vi "C-885 Chassis Engine.vi"() -> ()   [LabVIEW 2016]
uses:
  Stages Controls/Stage Notifier Element.ctl
  Stages Controls/Stage Actions.ctl
  Stages Controls/Stage Status.ctl
  C-885 Type Defs/C-885 Chassis Status.ctl
  PI GCS2 DLL/PI_GCS2_DLL_x64.dll
panel:
  in  "QUIT":bool
  in  "Abort":bool
  out "C-885 Found":bool
  out "Number Connected":i32
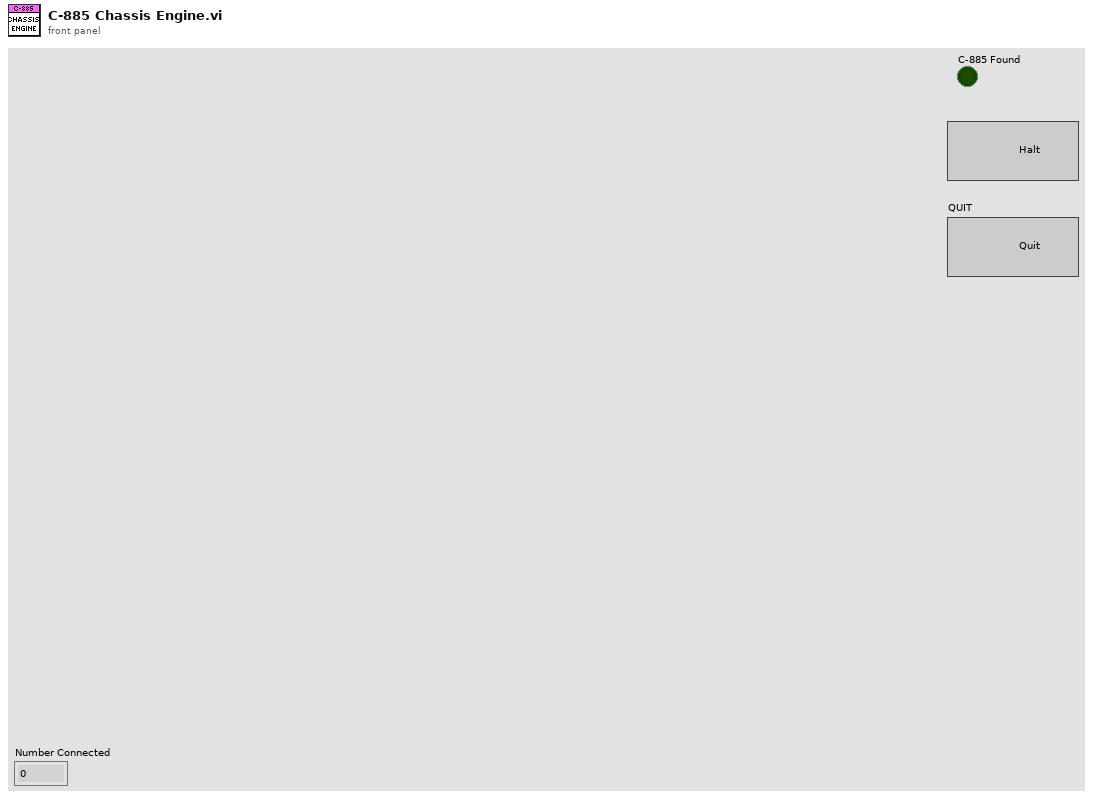
[diagram p1: front panel]
types:
  T1 = typedef "C-885 Chassis Status.ctl" = enum16{"Avalible", "Busy", "Halt"}
  T2 = typedef "Stage Notifier Element.ctl" = cluster{"Action":T3, "Axis":bool[], "Setpoint":dbl[], "Velocity":dbl, "Cmd Recvd?":bool, "Position":dbl[], "Status":T4, "Misc":variant}
  T3 = typedef "Stage Actions.ctl" = enum16{"Get Position", "MVR", "MOVE", "HALT", "ONTARGET", "ERROR", "REFERENCE", "INIT", "VELOCITY", "STATUS", "EXIT", "HOME", "ZEROPOS", "NANOPOS", "ANALOG", "QUIT"}
  T4 = typedef "Stage Status.ctl" = enum16{"Error", "Abort", "Busy", "On Target"}
  T5 = enum32{"Invalid", "Standard", "Closed", "Hidden", "Minimized", "Maximized"}
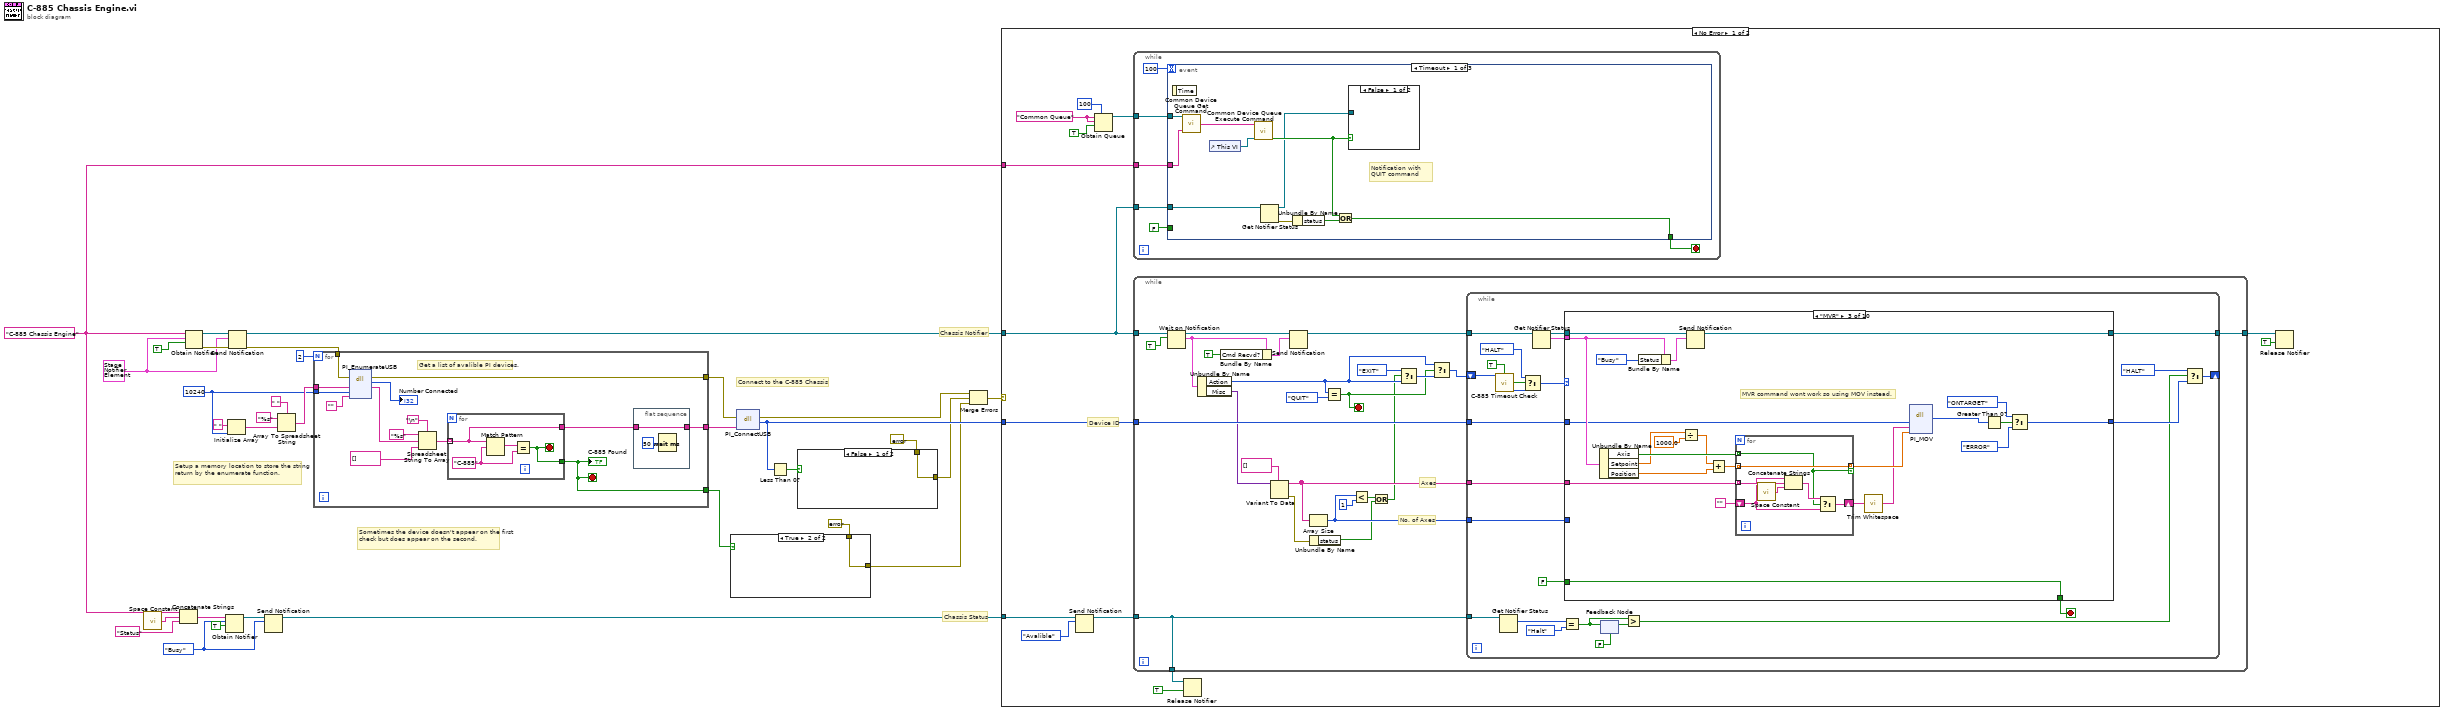
[diagram p0: block diagram]
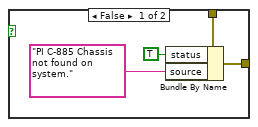
[diagram p2: hidden frame]
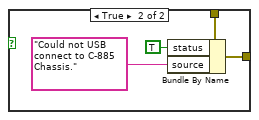
[diagram p3: hidden frame]
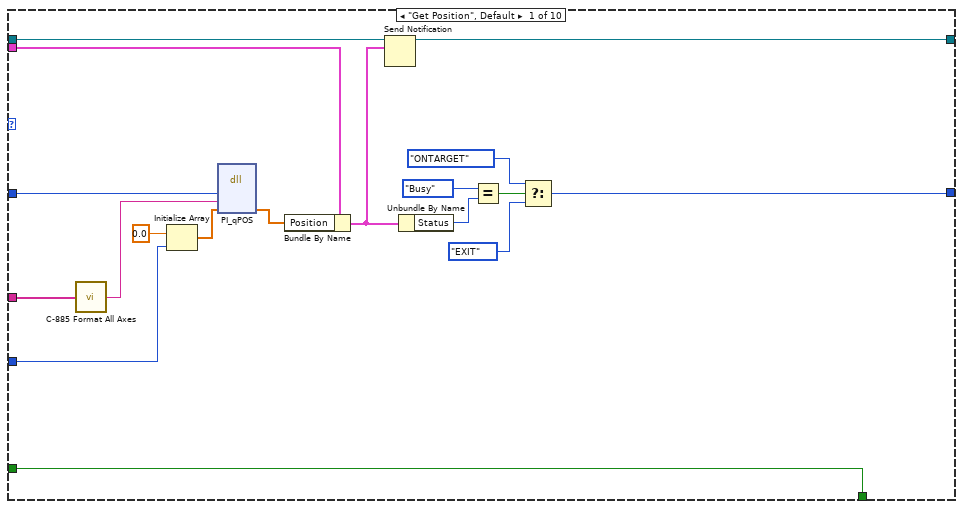
[diagram p4: hidden frame]
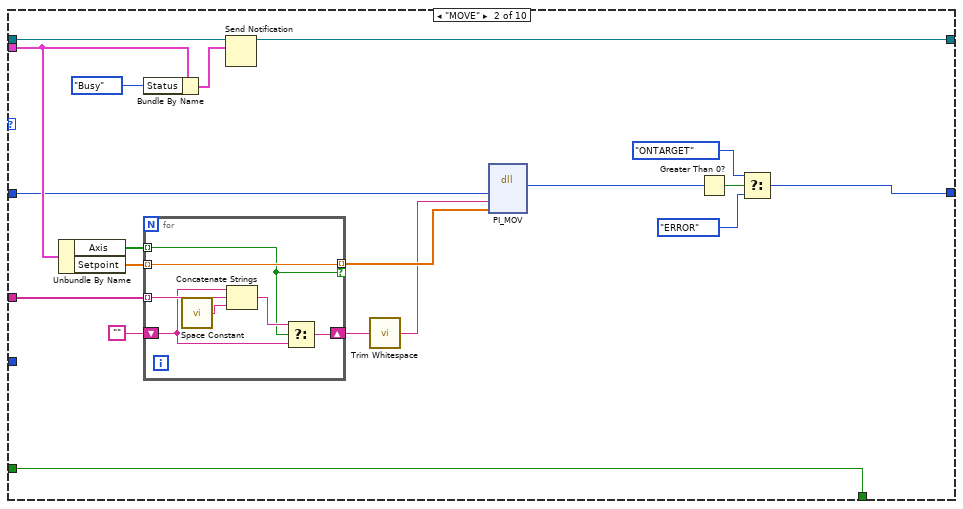
[diagram p5: hidden frame]
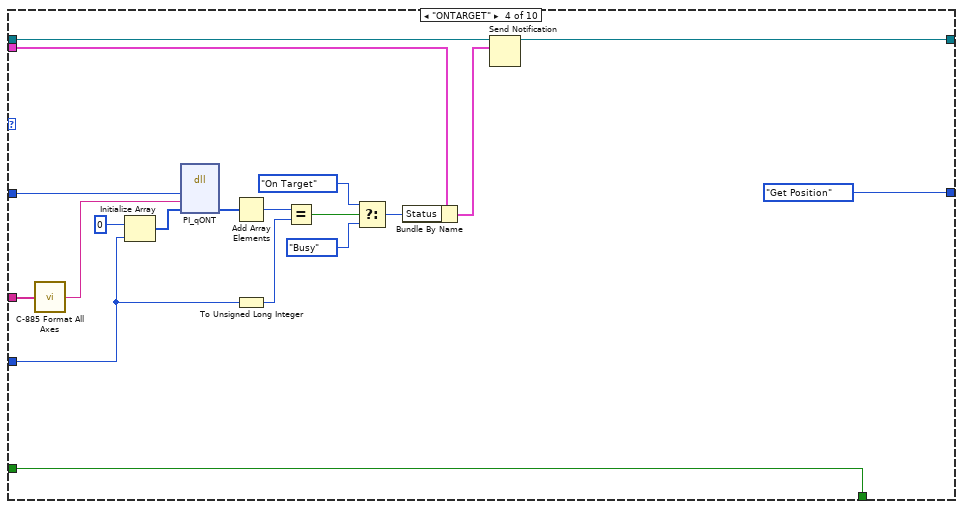
[diagram p6: hidden frame]
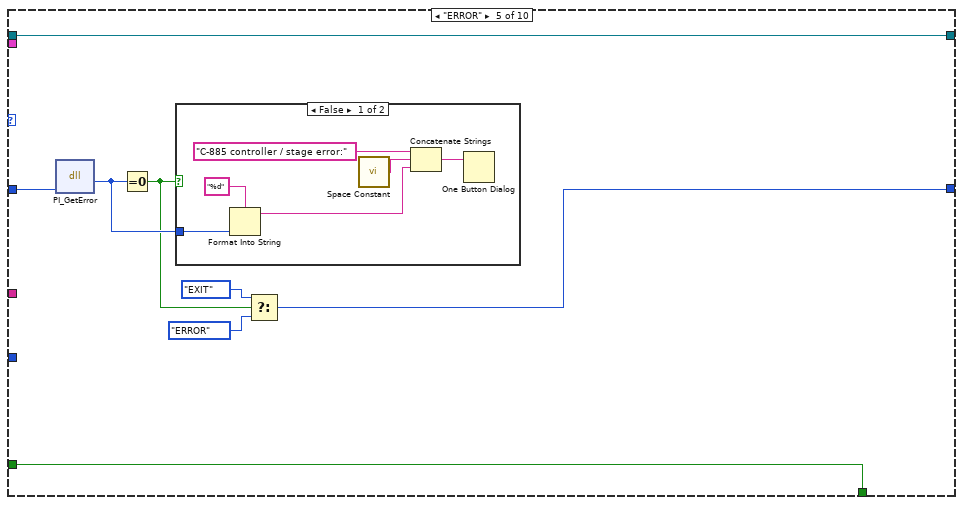
[diagram p7: hidden frame]
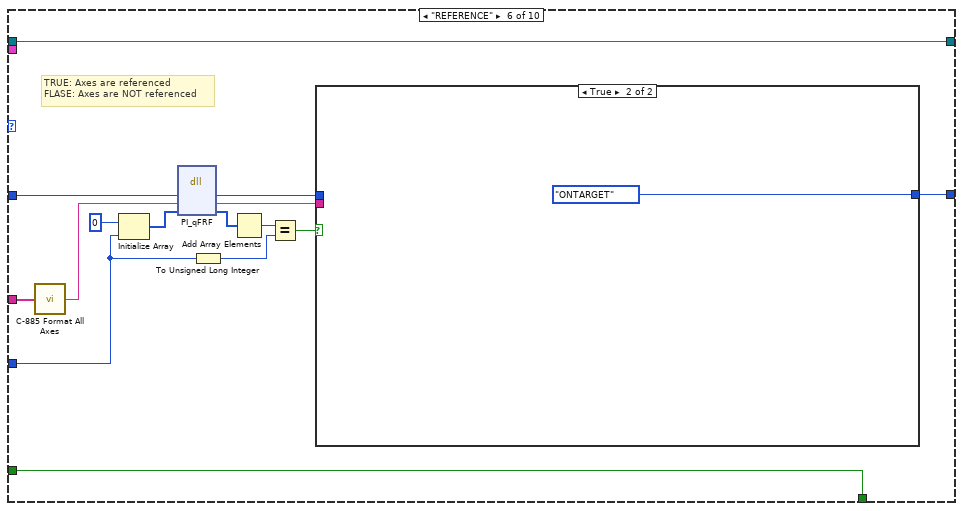
[diagram p9: hidden frame]
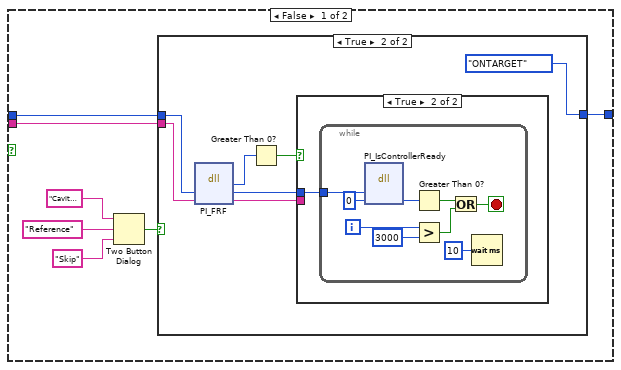
[diagram p10: hidden frame]
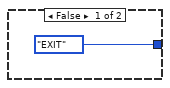
[diagram p11: hidden frame]
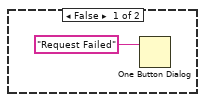
[diagram p12: hidden frame]
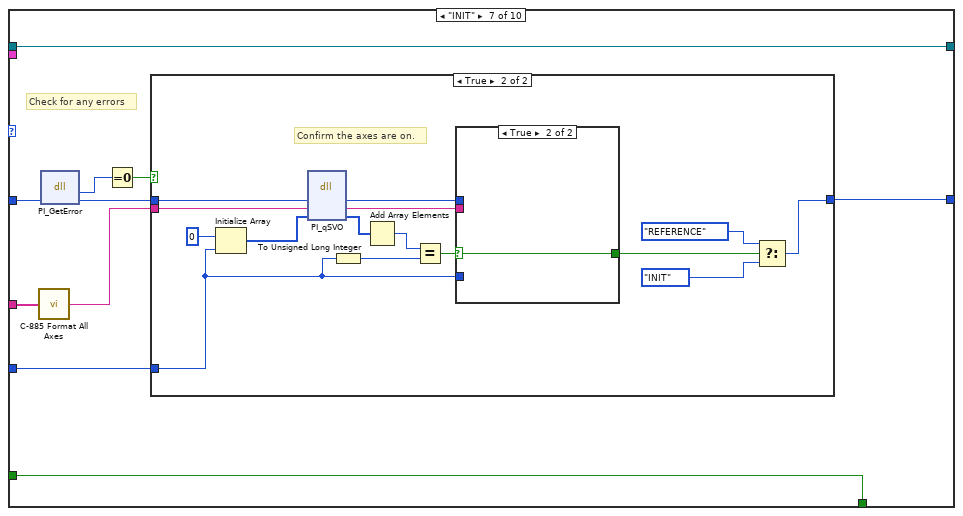
[diagram p13: hidden frame]
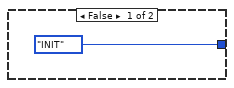
[diagram p14: hidden frame]
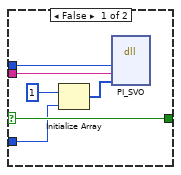
[diagram p15: hidden frame]
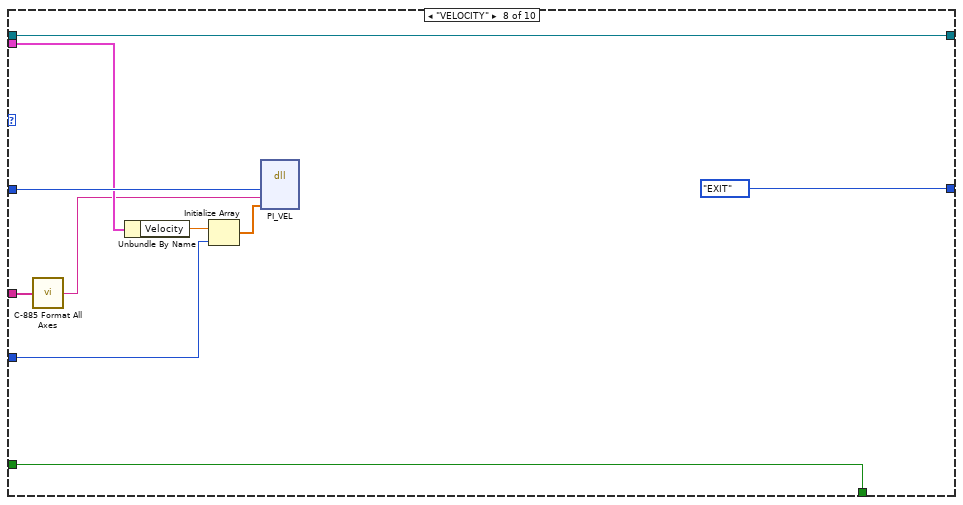
[diagram p16: hidden frame]
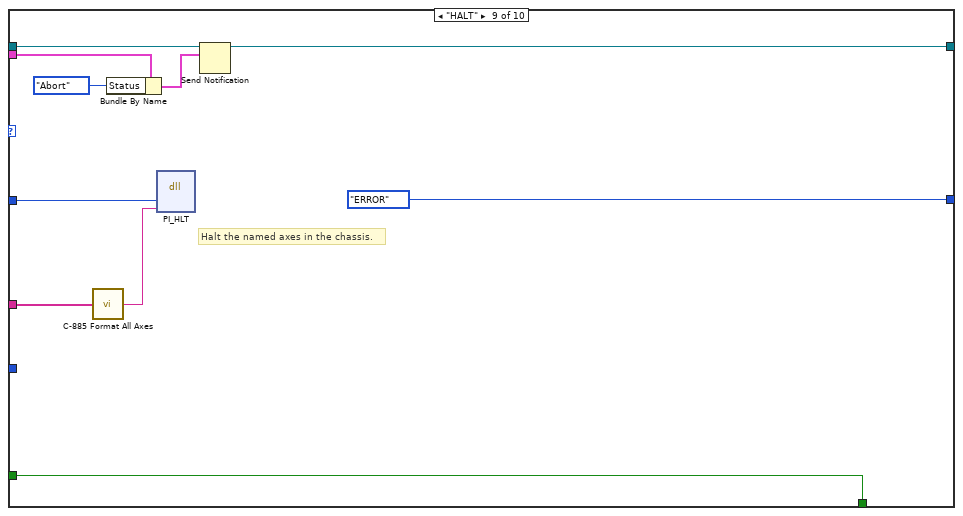
[diagram p17: hidden frame]
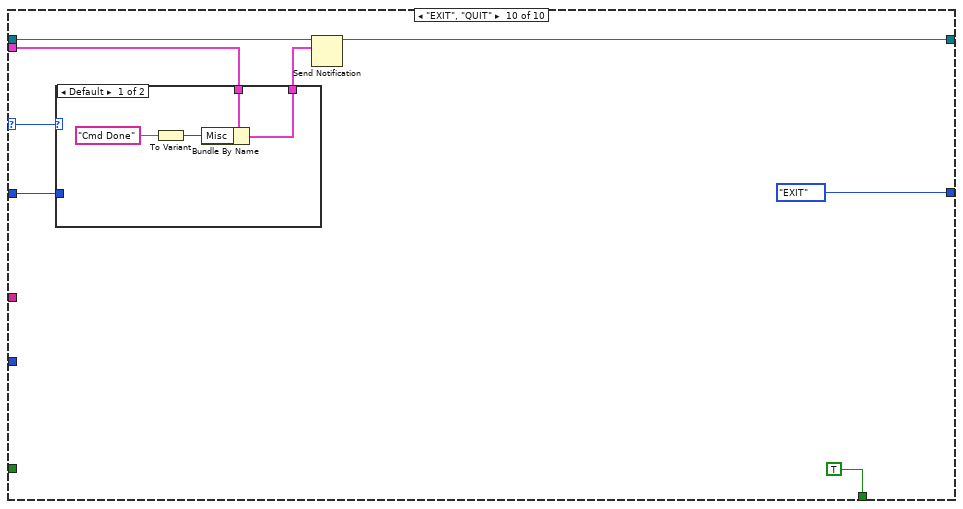
[diagram p18: hidden frame]
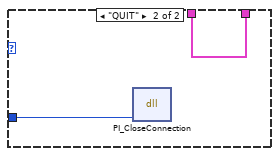
[diagram p19: hidden frame]
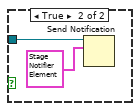
[diagram p20: hidden frame]
diagram:
  w6 = C-885_Chassis_Status."Busy" ("C-885 Chassis Status")
  w2 = T2 {"Action"=enum."Get Position", "Axis"=[], "Setpoint"=[], "Velocity"=0.5, "Cmd Recvd?"=FALSE, "Position"=[], "Status"=enum."Error", "Misc"=variant} ("Stage Status")
  w12 = "C-885 Chassis Engine" ("name (unnamed)")
  w27 = 10240 ("dimension size")
  # "Chassis Notifier"
  # "Chassis Status"
  # "Setup a memory location to store the string return by the enumerate function."
  # "Connect to the C-885 Chassis"
  # "Sometimes the device doesn't appear on the first check but does appear on the second."
  n1 = call <vilib>:"Space Constant.vi"() -> ("String"=w11:string)
  n2 = Concatenate Strings(w12, w11, "Status" ("name (unnamed)")) -> (w13:string)
  n3 = Obtain Notifier(name (unnamed)=w12, notification data type=w2, create if not found? (T)=TRUE) -> (notifier out=w5:refnum<notifier>, error out=w4:errorcluster)  [unwired: 1 in, 1 out]
  n4 = Obtain Notifier(name (unnamed)=w13, notification data type=w6, create if not found? (T)=TRUE) -> (notifier out=w8:refnum<notifier>)  [unwired: 1 in, 2 out]
  n5 = Initialize Array(" ", w27) -> (w31:string[])
  n6 = Send Notification(notification=w2, notifier=w5, error in (no error)=w4) -> (notifier out=w1:refnum<notifier>, error out=w3:errorcluster)
  n7 = Send Notification(notification=w6, notifier=w8) -> (notifier out=w7:refnum<notifier>)  [unwired: 1 in, 1 out]
  n8 = Array To Spreadsheet String(delimiter (Tab)=" ", array=w31, 3:"%s" ("format string")) -> (spreadsheet string=w28:string)
  n9 = for {
    N: 2 -> [_]
    tunnel: w28 -> [w41]
    tunnel: w27 -> [w40]
    tunnel: [w36] -> w25
    tunnel: [w35] -> w19
    tunnel: [w34] -> w24
    tunnel: w3 -> [w33]
    stop <- w35 stop-if-true
    # "Get a list of avalible PI devices."
    n10 = dll-call lib="C:/Users/George Sirinakis/Documents/Microscope-Control/Device Library/Stages/PI/PI GCS2 DLL/PI_GCS2_DLL_x64.dll" fn="PI_EnumerateUSB"(error in=w33, "szBuffer"=w41, "iBufferSize"=w40, "szFilter"="") -> (error out=w34:errorcluster, "return type"=→"Number Connected":i32, "szBuffer"=w38:string)  [unwired: 4 in, 1 out]
    n11 = Spreadsheet String To Array(delimiter (Tab)="\n", format string="%s", spreadsheet string=w38, array type (2D Dbl)=string[] []) -> (array=w43:string[])
    n12 = for {
      tunnel: w43 -> [w50] mode=indexing
      tunnel: [w50] -> w37
      tunnel: [w49] -> w35
      stop <- w49 stop-if-true
      w51 = "C-885"
      n13 = Match Pattern(string=w50, regular expression=w51) -> (match substring=w52:string)  [unwired: 1 in, 3 out]
      n14 = Equal?(x=w52, y=w51) -> (x = y?=w49:bool)
    }
    "C-885 Found" <- w35
    n15 = flat-sequence {
      tunnel: w37 -> [w48]
      tunnel: [w48] -> w36
      frame #0 {
        n16 = Wait (ms)(milliseconds to wait=u32 50) -> ()  [unwired: 1 out]
      }
    }
  }
  n17 = case shown="True" w19 {
    tunnel: errorcluster {"status"=FALSE, "code"=0, "source"=""} ("error in (no error)") -> [w54 w57]
    tunnel: [w53 w57] -> w15
    frame False {
      n18 = Bundle By Name(cluster=w54, "status"=TRUE, "source"="PI C-885 Chassis not found on system.") -> (w53:errorcluster)
    }
    frame True {
    }
  }
  n19 = dll-call lib="C:/Users/George Sirinakis/Documents/Microscope-Control/Device Library/Stages/PI/PI GCS2 DLL/PI_GCS2_DLL_x64.dll" fn="PI_ConnectUSB"(error in=w24, "szDescription"=w25) -> (error out=w17:errorcluster, "Device ID"=w22:i32)  [unwired: 3 in, 1 out]
  n20 = Less Than 0?(x=w22) -> (x < 0?=w21:bool)
  n21 = case shown="False" w21 {
    tunnel: errorcluster {"status"=FALSE, "code"=0, "source"=""} ("error in (no error)") -> [w58 w62]
    tunnel: [w58 w59] -> w16
    frame False {
    }
    frame True {
      n22 = Bundle By Name(cluster=w62, "status"=TRUE, "source"="Could not USB connect to C-885 Chassis.") -> (w59:errorcluster)
    }
  }
  n23 = Merge Errors(w17, w16, w15) -> (w14:errorcluster)
  n24 = case shown="No Error" w14 {
    selector: w14 -> [_ w380]
    tunnel: w1 -> [w70 w382]
    tunnel: w12 -> [w71 _]
    tunnel: w22 -> [w69 w381]
    tunnel: w7 -> [w65 w377]
    frame No Error {
      w75 = "Common Queue" ("Unique Notifier Name")
      # "Device ID"
      n25 = Send Notification(notification=C-885_Chassis_Status."Avalible", notifier=w65) -> (notifier out=w64:refnum<notifier>)  [unwired: 1 in, 1 out]
      n26 = Obtain Queue(max queue size (-1, unlimited)=100, name (unnamed)=w75, element data type=w75, create if not found? (T)=TRUE) -> (queue out=w72:refnum<queue>)  [unwired: 1 in, 2 out]
      n27 = while {
        tunnel: w70 -> [w346]
        tunnel: w72 -> [w345]
        tunnel: w71 -> [w344]
        stop <- w347 stop-if-true
        n28 = event shown="[0] Timeout" {
          selector: _ -> [_ _ _]
          dyn-events: _ -> [_ _ _]
          timeout: 100 -> [_ _ _]
          tunnel: [w352 w361 w370] -> w347
          tunnel: w346 -> [w358 _ w373]
          tunnel: w345 -> [w354 _ _]
          tunnel: w344 -> [w349 _ _]
          tunnel: FALSE -> [_ w361 w370]
          event Timeout {
            # "Notification with QUIT command"
            n29 = event-data() -> ()  [unwired: 1 in, 1 out]
            n30 = call "Common Device Queue Get Command.vi"("Common Queue"=w354, "Notifier Name"=w349) -> ("Command"=w355:string)  [unwired: 12 in, 1 out]
            n31 = control-ref of="This VI"() -> (w356:refnum<vi>)
            n32 = call "Common Device Queue Execute Command.vi"("Common Command"=w355, "VI Refnum"=w356) -> ("Quit?"=w351:bool)  [unwired: 12 in, 1 out]
            n33 = Get Notifier Status(notifier=w358) -> (notifier out=w350:refnum<notifier>, error out=w357:errorcluster)  [unwired: 1 in, 3 out]
            n34 = Unbundle By Name(w357) -> ("status"=w353:bool)
            n35 = Or(x=w351, y=w353) -> (x .or. y?=w352:bool)
            n36 = case shown="False" w351 {
              tunnel: w350 -> [_ w360]
              frame False {
              }
              frame True {
                n37 = Send Notification(notification=T2 {"Action"=enum."QUIT", "Axis"=[], "Setpoint"=[], "Velocity"=0.5, "Cmd Recvd?"=FALSE, "Position"=[], "Status"=enum."Error", "Misc"=variant} ("Stage Status"), notifier=w360) -> ()  [unwired: 1 in, 2 out]
              }
            }
          }
          event Application Instance Close? {
            n38 = event-data() -> ()  [unwired: 1 in, 5 out]
            n39 = control-ref of="This VI"() -> (w363:refnum<vi>)
            n40 = invoke class="VI" method="FP.Open"(reference=w363, "Activate"=TRUE ("Activate?"), "State"=T5."Standard") -> ()  [unwired: 2 in, 5 out]
            n41 = event-data("Discard?"=TRUE) -> ()  [unwired: 1 in, 1 out]
          }
          event "QUIT", "Abort": Value Change {
            n42 = event-data() -> ("CtlRef"=w372:refnum<vi>)  [unwired: 1 in]
            n43 = property class="Bool"(reference=w372) -> ("Label.Text"=w371:string)  [unwired: 1 in, 2 out]
            n44 = case shown="\"Default\", Default" w371 {
              tunnel: [Stage_Actions."EXIT" ("Action") Stage_Actions."QUIT" ("Action") Stage_Actions."HALT" ("Action")] -> w369
              frame "Default", Default {
              }
              frame "QUIT" {
              }
              frame "Abort" {
              }
            }
            n45 = Get Notifier Status(notifier=w373) -> (notifier out=w367:refnum<notifier>, current notification=w366:T2)  [unwired: 1 in, 3 out]
            n46 = Bundle By Name(cluster=w366, "Action"=w369) -> (w368:T2)
            n47 = Send Notification(notification=w368, notifier=w367) -> ()  [unwired: 1 in, 2 out]
          }
        }
      }
      n48 = while {
        tunnel: w70 -> [w100]
        tunnel: w69 -> [w99]
        tunnel: [w93] -> w68
        tunnel: w64 -> [w77]
        tunnel: [w77] -> w67
        stop <- w84 stop-if-true
        # "No. of Axes"
        # "Axes"
        n49 = Wait on Notification(notifier=w100, ignore previous (F)=TRUE) -> (notifier out=w98:refnum<notifier>, notification=w96:T2)  [unwired: 2 in, 2 out]
        n50 = Unbundle By Name(w96) -> ("Action"=w82:T3, "Misc"=w91:variant)
        n51 = Bundle By Name(cluster=w96, "Cmd Recvd?"=TRUE) -> (w94:T2)
        n52 = Variant To Data(type=string[] [], Variant=w91) -> (data=w89:string[], error out=w81:errorcluster)  [unwired: 1 in]
        n53 = Send Notification(notification=w94, notifier=w98) -> (notifier out=w97:refnum<notifier>)  [unwired: 1 in, 1 out]
        n54 = Array Size(array=w89) -> (size(s)=w87:i32)
        n55 = Unbundle By Name(w81) -> ("status"=w79:bool)
        n56 = Equal?(x=w82, y=Stage_Actions."QUIT") -> (x = y?=w84:bool)
        n57 = Less?(x=w87, y=1) -> (x < y?=w80:bool)
        n58 = Or(x=w80, y=w79) -> (x .or. y?=w78:bool)
        n59 = Select(t=Stage_Actions."EXIT", s=w78, f=w82) -> (s? t:f=w85:T3)
        n60 = Select(t=w82, s=w84, f=w85) -> (s? t:f=w83:T3)
        n61 = while {
          tunnel: w99 -> [w124]
          tunnel: w97 -> [w121]
          shift-right: [w123] -> _
          shift-left: w83 -> [w117]
          tunnel: [w106] -> w93
          tunnel: w89 -> [w111]
          tunnel: w87 -> [w112]
          tunnel: w77 -> [w109]
          stop <- w125 stop-if-true
          n62 = call "C-885 Timeout Check.vi"("Action"=w117, "User Input?"=TRUE) -> ("Timeout?"=w116:bool, "Action (Dup)"=w115:T3)  [unwired: 12 in]
          n63 = Get Notifier Status(notifier=w109) -> (current notification=w108:T1)  [unwired: 1 in, 4 out]
          n64 = Select(t=Stage_Actions."HALT" ("y"), s=w116, f=w115) -> (s? t:f=w114:T3)
          n65 = Get Notifier Status(notifier=w121) -> (notifier out=w120:refnum<notifier>, current notification=w119:T2)  [unwired: 1 in, 3 out]
          n66 = Equal?(x=w108, y=C-885_Chassis_Status."Halt" ("C-885 Chassis Status")) -> (x = y?=w103:bool)
          n67 = case shown="\"MVR\"" w114 {
            selector: w114 -> [_ _ _ _ _ _ _ _ _ w334]
            tunnel: w120 -> [w129 w147 w178 w203 w227 w248 w279 w318 w326 w332]
            tunnel: FALSE -> [w141 w163 w193 w219 w226 w247 w283 w317 w319 _]
            tunnel: [w141 w163 w193 w219 w226 w247 w283 w317 w319 TRUE] -> w125
            tunnel: [w135 w159 w189 Stage_Actions."Get Position" ("y") w220 w243 w280 Stage_Actions."EXIT" ("y") Stage_Actions."ERROR" ("y") Stage_Actions."EXIT" ("y")] -> w122
            tunnel: w124 -> [w142 w156 w186 w218 w225 w246 w285 w316 w328 w335]
            tunnel: [w127 w145 w176 w201 w227 w248 w279 w318 w324 w330] -> w106
            tunnel: w119 -> [w134 w157 w187 w209 _ _ _ w315 w327 w333]
            tunnel: w112 -> [w133 _ _ w213 _ w239 w276 w311 _ _]
            tunnel: w111 -> [w131 w152 w183 w205 _ w235 w278 w313 w322 _]
            frame "Get Position", Default {
              n68 = call "C-885 Format All Axes.vi"("All Axis Array"=w131) -> ("All Axes String"=w130:string)  [unwired: 14 in]
              n69 = Initialize Array(0.0 ("element"), w133) -> (w144:dbl[])
              n70 = dll-call lib="C:/Users/George Sirinakis/Documents/Microscope-Control/Device Library/Stages/PI/PI GCS2 DLL/PI_GCS2_DLL_x64.dll" fn="PI_qPOS"("Device ID"=w142, "szAxes"=w130, "pdValueArray"=w144) -> ("pdValueArray"=w132:dbl[])  [unwired: 6 in, 2 out]
              n71 = Bundle By Name(cluster=w134, "Position"=w132) -> (w128:T2)
              n72 = Send Notification(notification=w128, notifier=w129) -> (notifier out=w127:refnum<notifier>)  [unwired: 1 in, 1 out]
              n73 = Unbundle By Name(w128) -> ("Status"=w140:T4)
              n74 = Equal?(x=Stage_Status."Busy", y=w140) -> (x = y?=w138:bool)
              n75 = Select(t=Stage_Actions."ONTARGET" ("y"), s=w138, f=Stage_Actions."EXIT" ("y")) -> (s? t:f=w135:T3)
            }
            frame "MOVE" {
              n76 = Unbundle By Name(w157) -> ("Axis"=w154:bool[], "Setpoint"=w153:dbl[])
              n77 = Bundle By Name(cluster=w157, "Status"=Stage_Status."Busy") -> (w146:T2)
              n78 = for {
                tunnel: w154 -> [w166] mode=indexing
                tunnel: w153 -> [w167] mode=indexing
                tunnel: w152 -> [w170] mode=indexing
                shift-right: [w165] -> w149
                shift-left: "" -> [w164]
                tunnel: [w167] -> w150 mode=indexing if=w166
                n79 = call <vilib>:"Space Constant.vi"() -> ("String"=w169:string)
                n80 = Concatenate Strings(w164, w170, w169) -> (w168:string)
                n81 = Select(t=w168, s=w166, f=w164) -> (s? t:f=w165:string)
              }
              n82 = Send Notification(notification=w146, notifier=w147) -> (notifier out=w145:refnum<notifier>)  [unwired: 1 in, 1 out]
              n83 = call <vilib>:"Trim Whitespace.vi"("string"=w149) -> ("trimmed string"=w148:string)  [unwired: 1 in]
              n84 = dll-call lib="C:/Users/George Sirinakis/Documents/Microscope-Control/Device Library/Stages/PI/PI GCS2 DLL/PI_GCS2_DLL_x64.dll" fn="PI_MOV"("Device ID"=w156, "szAxes"=w148, "pdValueArray"=w150) -> ("Success"=w155:u8)  [unwired: 6 in, 2 out]
              n85 = Greater Than 0?(x=w155) -> (x > 0?=w162:bool)
              n86 = Select(t=Stage_Actions."ONTARGET" ("Action"), s=w162, f=Stage_Actions."ERROR" ("Action")) -> (s? t:f=w159:T3)
            }
            frame "MVR" {
              # "MVR command wont work so using MOV instead."
              n87 = Unbundle By Name(w187) -> ("Axis"=w184:bool[], "Setpoint"=w172:dbl[], "Position"=w175:dbl[])
              n88 = Bundle By Name(cluster=w187, "Status"=Stage_Status."Busy") -> (w177:T2)
              n89 = Divide(x=w172, y=1000.0) -> (x/y=w171:dbl[])
              n90 = Send Notification(notification=w177, notifier=w178) -> (notifier out=w176:refnum<notifier>)  [unwired: 1 in, 1 out]
              n91 = Add(x=w171, y=w175) -> (x+y=w174:dbl[])
              n92 = for {
                tunnel: w184 -> [w196] mode=indexing
                tunnel: w174 -> [w197] mode=indexing
                tunnel: w183 -> [w200] mode=indexing
                shift-right: [w195] -> w180
                shift-left: "" -> [w194]
                tunnel: [w197] -> w181 mode=indexing if=w196
                n93 = call <vilib>:"Space Constant.vi"() -> ("String"=w199:string)
                n94 = Concatenate Strings(w194, w200, w199) -> (w198:string)
                n95 = Select(t=w198, s=w196, f=w194) -> (s? t:f=w195:string)
              }
              n96 = call <vilib>:"Trim Whitespace.vi"("string"=w180) -> ("trimmed string"=w179:string)  [unwired: 1 in]
              n97 = dll-call lib="C:/Users/George Sirinakis/Documents/Microscope-Control/Device Library/Stages/PI/PI GCS2 DLL/PI_GCS2_DLL_x64.dll" fn="PI_MOV"("Device ID"=w186, "szAxes"=w179, "pdValueArray"=w181) -> ("Success"=w185:u8)  [unwired: 6 in, 2 out]
              n98 = Greater Than 0?(x=w185) -> (x > 0?=w192:bool)
              n99 = Select(t=Stage_Actions."ONTARGET" ("Action"), s=w192, f=Stage_Actions."ERROR" ("Action")) -> (s? t:f=w189:T3)
            }
            frame "ONTARGET" {
              n100 = call "C-885 Format All Axes.vi"("All Axis Array"=w205) -> ("All Axes String"=w204:string)  [unwired: 14 in]
              n101 = Initialize Array(u32 0 ("element"), w213) -> (w216:u32[])
              n102 = dll-call lib="C:/Users/George Sirinakis/Documents/Microscope-Control/Device Library/Stages/PI/PI GCS2 DLL/PI_GCS2_DLL_x64.dll" fn="PI_qONT"("Device ID"=w218, "szAxes"=w204, "pdValueArray"=w216) -> ("pdValueArray"=w215:u32[])  [unwired: 6 in, 2 out]
              n103 = Add Array Elements(numeric array=w215) -> (sum=w214:u32)
              n104 = To Unsigned Long Integer(number=w213) -> (unsigned 32bit integer=w212:u32)
              n105 = Equal?(x=w214, y=w212) -> (x = y?=w211:bool)
              n106 = Select(t=Stage_Status."On Target" ("Status"), s=w211, f=Stage_Status."Busy" ("Status")) -> (s? t:f=w206:T4)
              n107 = Bundle By Name(cluster=w209, "Status"=w206) -> (w202:T2)
              n108 = Send Notification(notification=w202, notifier=w203) -> (notifier out=w201:refnum<notifier>)  [unwired: 1 in, 1 out]
            }
            frame "ERROR" {
              n109 = dll-call lib="C:/Users/George Sirinakis/Documents/Microscope-Control/Device Library/Stages/PI/PI GCS2 DLL/PI_GCS2_DLL_x64.dll" fn="PI_GetError"("Device ID"=w225) -> ("Error Code"=w224:i32)  [unwired: 4 in, 2 out]
              n110 = Equal To 0?(x=w224) -> (x = 0?=w223:bool)
              n111 = case shown="False" w223 {
                tunnel: w224 -> [w231 _]
                frame False {
                  n112 = Format Into String(format string="%d", w231) -> (resulting string=w229:string)  [unwired: 2 in, 1 out]
                  n113 = call <vilib>:"Space Constant.vi"() -> ("String"=w232:string)
                  n114 = Concatenate Strings("C-885 controller / stage error:", w232, w229) -> (w228:string)
                  n115 = One Button Dialog(message=w228) -> ()  [unwired: 1 in, 1 out]
                }
                frame True {
                }
              }
              n116 = Select(t=Stage_Actions."EXIT", s=w223, f=Stage_Actions."ERROR" ("Action")) -> (s? t:f=w220:T3)
            }
            frame "REFERENCE" {
              # "TRUE: Axes are referenced\nFLASE: Axes are NOT referenced"
              n117 = call "C-885 Format All Axes.vi"("All Axis Array"=w235) -> ("All Axes String"=w234:string)  [unwired: 14 in]
              n118 = Initialize Array(u32 0 ("element"), w239) -> (w244:u32[])
              n119 = dll-call lib="C:/Users/George Sirinakis/Documents/Microscope-Control/Device Library/Stages/PI/PI GCS2 DLL/PI_GCS2_DLL_x64.dll" fn="PI_qFRF"("Device ID"=w246, "szAxes"=w234, "pdValueArray"=w244) -> ("Device ID"=w241:i32, "szAxes"=w242:string, "pdValueArray"=w240:u32[])  [unwired: 4 in, 2 out]
              n120 = To Unsigned Long Integer(number=w239) -> (unsigned 32bit integer=w237:u32)
              n121 = Add Array Elements(numeric array=w240) -> (sum=w238:u32)
              n122 = Equal?(x=w238, y=w237) -> (x = y?=w236:bool)
              n123 = case shown="True" w236 {
                tunnel: [w249 Stage_Actions."ONTARGET" ("Action")] -> w243
                tunnel: w242 -> [w250 _]
                tunnel: w241 -> [w251 _]
                frame False {
                  n124 = Two Button Dialog(message="Cavity stage (N-216) is not referenced.", 1:"Skip" ("F button name (\"Cancel\")"), 2:"Reference" ("T button name (\"OK\")")) -> (T button?=w252:bool)
                  n125 = case shown="True" w252 {
                    tunnel: w251 -> [_ w257]
                    tunnel: w250 -> [_ w258]
                    tunnel: [Stage_Actions."EXIT" ("Action") Stage_Actions."ONTARGET" ("Action")] -> w249
                    frame False {
                    }
                    frame True {
                      n126 = dll-call lib="C:/Users/George Sirinakis/Documents/Microscope-Control/Device Library/Stages/PI/PI GCS2 DLL/PI_GCS2_DLL_x64.dll" fn="PI_FRF"("Device ID"=w257, "szAxes"=w258) -> ("Success"=w259:u8, "Device ID"=w261:i32, "szAxes"=w262:string)  [unwired: 3 in, 2 out]
                      n127 = Greater Than 0?(x=w259) -> (x > 0?=w260:bool)
                      n128 = case shown="True" w260 {
                        tunnel: w261 -> [_ w265]
                        tunnel: w262 -> [_ _]
                        frame False {
                          n129 = One Button Dialog(message="Request Failed") -> ()  [unwired: 1 in, 1 out]
                        }
                        frame True {
                          n130 = while {
                            tunnel: w265 -> [w274]
                            i -> [w272]
                            stop <- w267 stop-if-true
                            n131 = dll-call lib="C:/Users/George Sirinakis/Documents/Microscope-Control/Device Library/Stages/PI/PI GCS2 DLL/PI_GCS2_DLL_x64.dll" fn="PI_IsControllerReady"("Device ID"=w274, "piControllerReady"=0) -> ("piControllerReady"=w270:i32)  [unwired: 5 in, 2 out]
                            n132 = Greater Than 0?(x=w270) -> (x > 0?=w269:bool)
                            n133 = Greater?(x=w272, y=3000) -> (0:w268:bool)
                            n134 = Or(x=w269, y=w268) -> (x .or. y?=w267:bool)
                            n135 = Wait (ms)(milliseconds to wait=u32 10) -> ()  [unwired: 1 out]
                          }
                        }
                      }
                    }
                  }
                }
                frame True {
                }
              }
            }
            frame "INIT" {
              # "Check for any errors"
              n136 = call "C-885 Format All Axes.vi"("All Axis Array"=w278) -> ("All Axes String"=w277:string)  [unwired: 14 in]
              n137 = dll-call lib="C:/Users/George Sirinakis/Documents/Microscope-Control/Device Library/Stages/PI/PI GCS2 DLL/PI_GCS2_DLL_x64.dll" fn="PI_GetError"("Device ID"=w285) -> ("Error Code"=w284:i32, "Device ID"=w281:i32)  [unwired: 3 in, 2 out]
              n138 = Equal To 0?(x=w284) -> (x = 0?=w282:bool)
              n139 = case shown="True" w282 {
                tunnel: w281 -> [_ w301]
                tunnel: w277 -> [_ w300]
                tunnel: [Stage_Actions."INIT" ("Action") w298] -> w280
                tunnel: w276 -> [_ w293]
                frame False {
                }
                frame True {
                  # "Confirm the axes are on."
                  n140 = Initialize Array(u32 0 ("element"), w293) -> (w295:u32[])
                  n141 = dll-call lib="C:/Users/George Sirinakis/Documents/Microscope-Control/Device Library/Stages/PI/PI GCS2 DLL/PI_GCS2_DLL_x64.dll" fn="PI_qSVO"("Device ID"=w301, "szAxes"=w300, "pdValueArray"=w295) -> ("Device ID"=w291:i32, "szAxes"=w292:string, "pdValueArray"=w290:u32[])  [unwired: 4 in, 2 out]
                  n142 = To Unsigned Long Integer(number=w293) -> (unsigned 32bit integer=w287:u32)
                  n143 = Add Array Elements(numeric array=w290) -> (sum=w289:u32)
                  n144 = Equal?(x=w289, y=w287) -> (x = y?=w288:bool)
                  n145 = case shown="True" w288 {
                    selector: w288 -> [w305 w308]
                    tunnel: w292 -> [w306 _]
                    tunnel: w291 -> [w307 _]
                    tunnel: [w305 w308] -> w299
                    tunnel: w293 -> [w303 _]
                    frame False {
                      n146 = Initialize Array(u32 1 ("element"), w303) -> (w302:u32[])
                      n147 = dll-call lib="C:/Users/George Sirinakis/Documents/Microscope-Control/Device Library/Stages/PI/PI GCS2 DLL/PI_GCS2_DLL_x64.dll" fn="PI_SVO"("Device ID"=w307, "szAxes"=w306, "pdValueArray"=w302) -> ()  [unwired: 7 in, 2 out]
                    }
                    frame True {
                    }
                  }
                  n148 = Select(t=Stage_Actions."REFERENCE" ("Action"), s=w299, f=Stage_Actions."INIT" ("Action")) -> (s? t:f=w298:T3)
                }
              }
            }
            frame "VELOCITY" {
              n149 = call "C-885 Format All Axes.vi"("All Axis Array"=w313) -> ("All Axes String"=w309:string)  [unwired: 14 in]
              n150 = Unbundle By Name(w315) -> ("Velocity"=w312:dbl)
              n151 = Initialize Array(w312, w311) -> (w310:dbl[])
              n152 = dll-call lib="C:/Users/George Sirinakis/Documents/Microscope-Control/Device Library/Stages/PI/PI GCS2 DLL/PI_GCS2_DLL_x64.dll" fn="PI_VEL"("Device ID"=w316, "szAxes"=w309, "pdValueArray"=w310) -> ()  [unwired: 7 in, 2 out]
            }
            frame "HALT" {
              # "Halt the named axes in the chassis."
              n153 = call "C-885 Format All Axes.vi"("All Axis Array"=w322) -> ("All Axes String"=w320:string)  [unwired: 14 in]
              n154 = Bundle By Name(cluster=w327, "Status"=Stage_Status."Abort") -> (w325:T2)
              n155 = dll-call lib="C:/Users/George Sirinakis/Documents/Microscope-Control/Device Library/Stages/PI/PI GCS2 DLL/PI_GCS2_DLL_x64.dll" fn="PI_HLT"("Device ID"=w328, "szAxes"=w320) -> ()  [unwired: 6 in, 2 out]
              n156 = Send Notification(notification=w325, notifier=w326) -> (notifier out=w324:refnum<notifier>)  [unwired: 1 in, 1 out]
            }
            frame "EXIT", "QUIT" {
              n157 = case shown="Default" w334 {
                tunnel: w335 -> [_ w341]
                tunnel: w333 -> [w340 w342]
                tunnel: [w337 w342] -> w331
                frame Default {
                  n158 = To Variant(anything="Cmd Done") -> (Variant=w338:variant)
                  n159 = Bundle By Name(cluster=w340, "Misc"=w338) -> (w337:T2)
                }
                frame "QUIT" {
                  n160 = dll-call lib="C:/Users/George Sirinakis/Documents/Microscope-Control/Device Library/Stages/PI/PI GCS2 DLL/PI_GCS2_DLL_x64.dll" fn="PI_CloseConnection"("Device ID"=w341) -> ()  [unwired: 5 in, 2 out]
                }
              }
              n161 = Send Notification(notification=w331, notifier=w332) -> (notifier out=w330:refnum<notifier>)  [unwired: 1 in, 1 out]
            }
          }
          n162 = feedback #1(FALSE) -> (w104:bool)
          n163 = feedback-in #1(w103) -> ()
          n164 = Greater?(x=w103, y=w104) -> (0:w102:bool)
          n165 = Select(t=Stage_Actions."HALT", s=w102, f=w122) -> (s? t:f=w123:T3)
        }
      }
      n166 = Release Notifier(notifier=w67, force destroy? (F)=TRUE) -> ()  [unwired: 1 in, 3 out]
      n167 = Release Notifier(notifier=w68, force destroy? (F)=TRUE) -> ()  [unwired: 1 in, 3 out]
    }
    frame Error {
      n168 = Release Notifier(notifier=w377, force destroy? (F)=TRUE) -> ()  [unwired: 1 in, 3 out]
      n169 = dll-call lib="C:/Users/George Sirinakis/Documents/Microscope-Control/Device Library/Stages/PI/PI GCS2 DLL/PI_GCS2_DLL_x64.dll" fn="PI_CloseConnection"(error in=w380, "Device ID"=w381) -> (error out=w379:errorcluster)  [unwired: 4 in, 1 out]
      n170 = Release Notifier(notifier=w382, force destroy? (F)=TRUE, error in (no error)=w379) -> (error out=w387:errorcluster)  [unwired: 2 out]
      n171 = Unbundle By Name(w387) -> ("source"=w384:string)
      n172 = Concatenate Strings("C-885 Initialization Error", "\r", w384) -> (w383:string)
      n173 = One Button Dialog(message=w383) -> ()  [unwired: 1 in, 1 out]
    }
  }
